vi "Write Control Refnum.vi"(8 "error in (no error)":errorcluster, 10 "Ctl Refnum":refnum<vi>, 11 "UI-Bus_Boolean in":refnum<class "UI-Bus_Extended.lvclass">) -> (0 "error out":errorcluster, 3 "UI-Bus_Boolean out":refnum<class "UI-Bus_Extended.lvclass">)   [LabVIEW 2021, in "UI-Bus_Extended.lvclass"]
uses:
  UI-Bus_Extended.lvclass
  UI-Bus_Extended.lvclass/UI-Bus_Extended.ctl
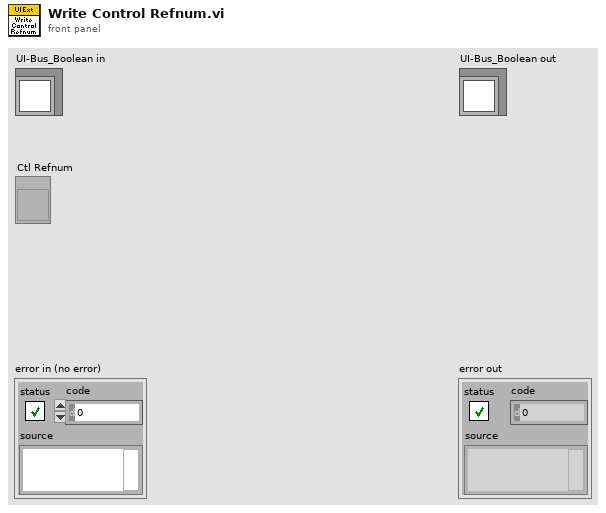
[diagram p1: front panel]
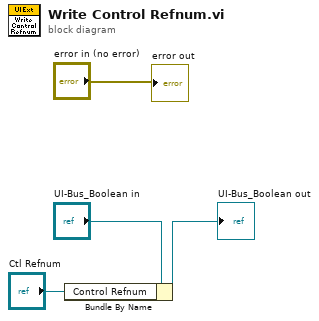
[diagram p0: block diagram]
diagram:
  n1 = Bundle By Name(cluster="UI-Bus_Boolean in", "Control Refnum"="Ctl Refnum") -> (→"UI-Bus_Boolean out":refnum<class "UI-Bus_Extended.lvclass">)
  "error out" <- "error in (no error)"
